vi "Esercitazione 5 - Esercizio per casa, Array Palindromo.vi"() -> ()   [LabVIEW 2018]
panel:
  in  "Array":dbl[](array[numeric])
  out "Boolean":bool
  # "dato un array qualsiasi, determinare se è palindromo"
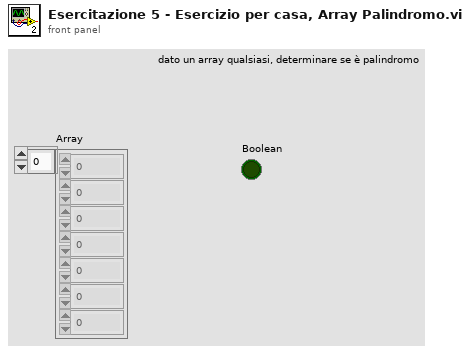
[diagram p1: front panel]
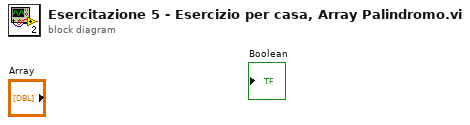
[diagram p0: block diagram]
diagram:
